vi "SequenceIndexGet.vi"(8 "error in (no error)":errorcluster, 10 "SequenceIndexName":string, 11 "VariableManagerRef in":refnum<vi>) -> (0 "error out":errorcluster, 2 "SequenceIndex":refnum<class "SequenceIndex.lvclass">, 3 "VariableManagerRef out":refnum<vi>)   [LabVIEW 2013, in "VariableManagerAPI.lvlib"]
doc: "Return sequence index definition of SequenceIndexName\n\nAn error is thrown if a SequenceIndexName does not exist."
uses:
  VariableManagerAPI.lvlib
  VariableManager/VariableManager.lvclass
  SequenceIndex/SequenceIndex.lvclass
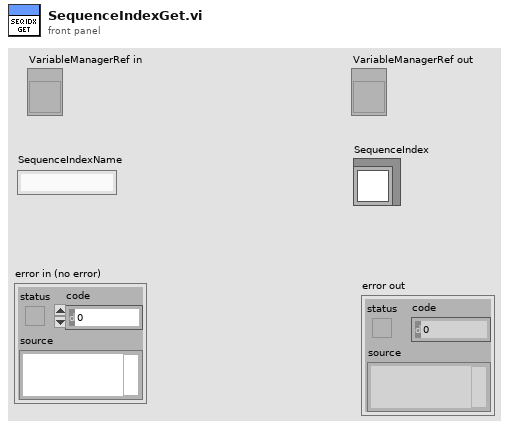
[diagram p1: front panel]
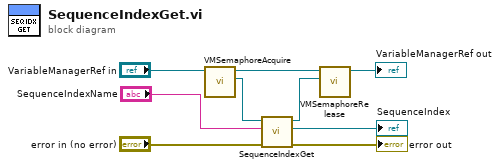
[diagram p0: block diagram]
diagram:
  n1 = call "VMSemaphoreAcquire.vi"("VariableManagerRef in"="VariableManagerRef in") -> ("VariableManager"=w6:refnum<class "VariableManager.lvclass">, "VariableManagerRef out"=w8:refnum<vi>)  [unwired: 7 in, 2 out]
  n2 = call-dynamic "SequenceIndexGet.vi"("error in (no error)"="error in (no error)", "SequenceIndexName"="SequenceIndexName", "VariableManager in"=w6) -> ("error out"=→"error out":errorcluster, "SequenceIndex"=→"SequenceIndex":refnum<class "SequenceIndex.lvclass">, "VariableManager out"=w5:refnum<class "VariableManager.lvclass">)  [unwired: 6 in]
  n3 = call "VMSemaphoreRelease.vi"("VariableManager"=w5, "VariableManagerRef in"=w8) -> ("VariableManagerRef out"=→"VariableManagerRef out":refnum<vi>)  [unwired: 8 in, 1 out]
